vi "Corr Transducers Build Meas Paths.vi"(0 "transducer":T1={"Path"=path "", "Ratio:"="", "Name:"="", "btn rem"=FALSE, "btn up"=FALSE, "btn down"=FALSE, "s.n.:"="", "btn open"=FALSE, "ratio o/i"=1.0, "chn hi"=0, "chn lo"=0, "Phase index"=1} {"Phase index" min=1 step=1}, 1 "measurement folder root path":path, 2 "transducer index":i32) -> (3 "destination folder full path":path, 4 "destination relative folder path":string, 5 "destination header full path":path, 6 "destination header realtive path":string)   [LabVIEW 2013]
doc: "The VI takes single transducer and new measurement root path and builds paths of the transducer as it will be stored in the new measurement folder."
uses:
  Corr Tranducer Item.ctl
panel:
  # "ADC:"
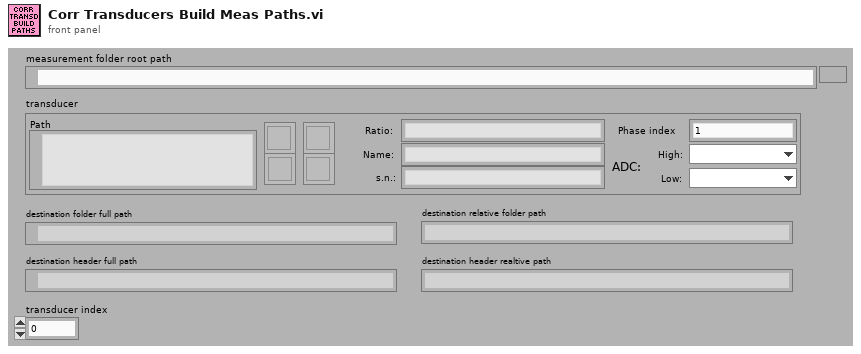
[diagram p1: front panel]
types:
  T1 = typedef "Corr Tranducer Item.ctl" = cluster{"Path":path, "Ratio:":string, "Name:":string, "btn rem":bool, "btn up":bool, "btn down":bool, "s.n.:":string, "btn open":bool, "ratio o/i":dbl, "chn hi":u16, "chn lo":u16, "Phase index":i32}
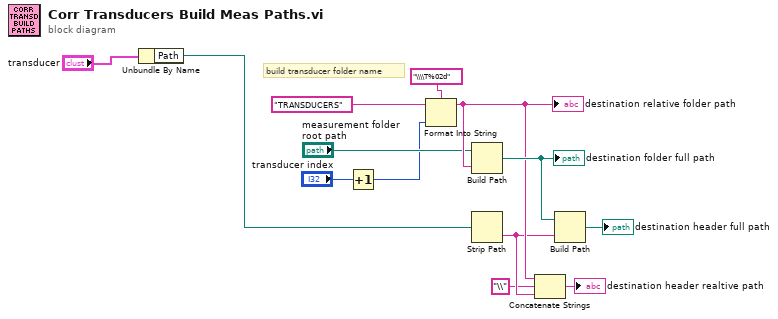
[diagram p0: block diagram]
diagram:
  # "build transducer folder name"
  n1 = Unbundle By Name("transducer") -> ("Path"=w10:path)
  n2 = Increment(x="transducer index") -> (x+1=w1:i32)
  n3 = Format Into String(format string="\\\\T%02d", initial string="TRANSDUCERS" ("name or relative path"), w1) -> (resulting string=w8:string)  [unwired: 1 in, 1 out]
  "destination relative folder path" <- w8
  n4 = Build Path(base path="measurement folder root path", name or relative path=w8) -> (appended path=w11:path)
  "destination folder full path" <- w11
  n5 = Strip Path(path=w10) -> (name=w7:string)  [unwired: 1 out]
  n6 = Concatenate Strings(w8, "\\" ("string"), w7) -> (→"destination header realtive path":string)
  n7 = Build Path(base path=w11, name or relative path=w7) -> (appended path=→"destination header full path":path)
